vi "GLdrv_TRIG_COND_SOUR.vi"(0 "Connection ID":T2, 5 "COND":i32=1 min=0 max=1, 7 "Source":T1(ring), 9 "Alarm Time or Date":string, 11 "error in (no error)":errorcluster, 12 "Week":u8 format="%08b", 13 "Query(f)":bool) -> (4 "Connection ID Out":T2, 8 "Source out":T1(ring), 10 "Alarm Time or Date out":string, 14 "Week out":u8 format="%08b", 15 "error out":errorcluster)   [LabVIEW 2017, in "GL860_Driver.lvlib"]
doc: "トリガを検知する種類を設定します\nOff：　トリガを検知しません\nAMP: 指定ﾚﾍﾞﾙでトリガを検知します(CH,LOGIC,PULSEで設定)\nALAR：　アラーム発生でトリガを検知します。\nDATE：　指定時刻でトリガを検知します。(繰り返しOFF時に有効です)\n例）:TRIG:COND0:DATE,\"2010-01-01 00:00:00”\nLDATE：　指定時間でトリガを検知します。(繰り返しON時に有効です)\n例）:TRIG:COND1:LDATE,\"12:34:56”\nWEEK: 曜日と時間でトリガを検知します。\n<曜日設定> ０１２３４５６７ (8bit) 0=Off/1=On\n日月火水木金土\n例）　:TRIG:COND0:SOUR WEEK,127,\"12:34:56”\nEXTernal: 外部信号でトリガを検知します\nTIME: 時間経過(秒)でトリガを検知します(指定時間経過したら開始ま\nたは停止します。）\n例）　:TRIG:COND1:SOUR TIME,6000 (ストップトリガを100分後に設\n定します)"
uses:
  GL860_Driver.lvlib
  ConnectionID.ctl
  GLdrv_RW.ctl
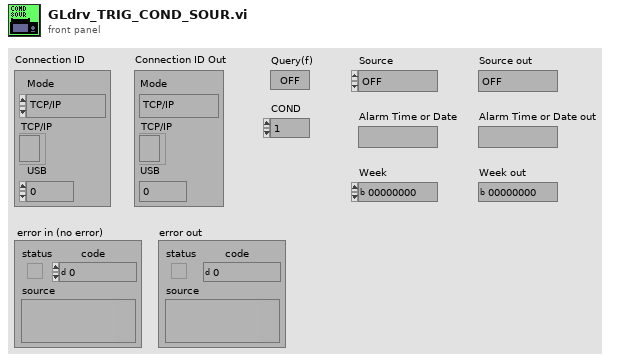
[diagram p1: front panel]
types:
  T1 = enum16{"OFF", "AMP", "ALAR", "DATE", "LDATE", "WEEK", "EXT", "TIME"}
  T2 = typedef "ConnectionID.ctl" = cluster{"Mode":enum16{"TCP/IP", "USB"}, "TCP/IP":refnum<k5>, "USB":i32}
  T3 = typedef "GLdrv_RW.ctl" = enum16{"Auto", "Read", "Write", "Buffer"}
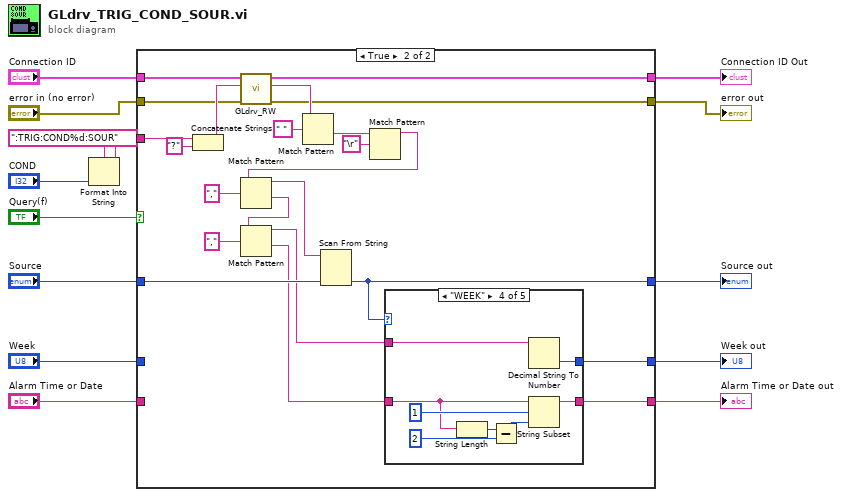
[diagram p0: block diagram]
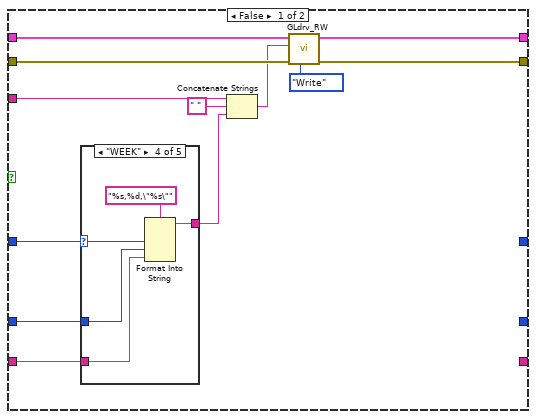
[diagram p2: hidden frame]
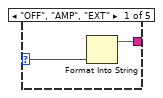
[diagram p3: hidden frame]
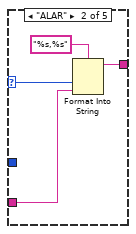
[diagram p4: hidden frame]
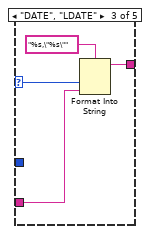
[diagram p5: hidden frame]
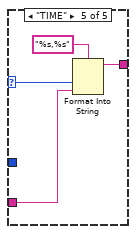
[diagram p6: hidden frame]
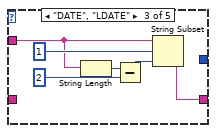
[diagram p9: hidden frame]
diagram:
  n1 = Format Into String(format string=":TRIG:COND%d:SOUR" ("Command"), "COND") -> (resulting string=w9:string)  [unwired: 2 in, 1 out]
  n2 = case shown="TRUE" "Query(f)" {
    tunnel: w9 -> [w26 w64]
    tunnel: [w21 w57] -> w14
    tunnel: [w23 w61] -> w13
    tunnel: "Connection ID" -> [w24 w62]
    tunnel: "error in (no error)" -> [w22 w58]
    tunnel: "Source" -> [w15 w56]
    tunnel: [_ w50] -> w6
    tunnel: "Alarm Time or Date" -> [w17 _]
    tunnel: "Week" -> [w16 _]
    tunnel: [_ w49] -> w3
    tunnel: [_ w47] -> w2
    frame False {
      n3 = case shown="\"WEEK\"" w15 {
        selector: w15 -> [w27 w31 w35 w40 w44]
        tunnel: [w28 w32 w36 w41 w45] -> w18
        tunnel: w17 -> [_ w29 w33 w38 w42]
        tunnel: w16 -> [_ _ _ w37 _]
        frame "OFF", "AMP", "EXT" {
          n4 = Format Into String(w27) -> (resulting string=w28:string)  [unwired: 3 in, 1 out]
        }
        frame "ALAR" {
          n5 = Format Into String(format string="%s,%s", w31, w29) -> (resulting string=w32:string)  [unwired: 2 in, 1 out]
        }
        frame "DATE", "LDATE" {
          n6 = Format Into String(format string="%s,\"%s\"", w35, w33) -> (resulting string=w36:string)  [unwired: 2 in, 1 out]
        }
        frame "WEEK" {
          n7 = Format Into String(format string="%s,%d,\"%s\"", w40, w37, w38) -> (resulting string=w41:string)  [unwired: 2 in, 1 out]
        }
        frame "TIME" {
          n8 = Format Into String(format string="%s,%s", w44, w42) -> (resulting string=w45:string)  [unwired: 2 in, 1 out]
        }
      }
      n9 = Concatenate Strings(w26, " " ("string"), w18) -> (w20:string)
      n10 = call "GLdrv_RW.vi"("Mode(read)"=GLdrv_RW."Write", "error in (no error)"=w22, "data in"=w20, "Connection ID"=w24) -> ("error out"=w21:errorcluster, "Connection ID Out"=w23:T2)  [unwired: 3 in, 3 out]
    }
    frame True {
      n11 = Concatenate Strings(w64, "?" ("string")) -> (w60:string)
      n12 = call "GLdrv_RW.vi"("error in (no error)"=w58, "data in"=w60, "Connection ID"=w62) -> ("error out"=w57:errorcluster, "data out"=w59:string, "Connection ID Out"=w61:T2)  [unwired: 4 in, 2 out]
      n13 = Match Pattern(string=w59, regular expression=" " ("search string/char (-)")) -> (after substring=w65:string)  [unwired: 4 out]
      n14 = Match Pattern(string=w65, regular expression="\r") -> (before substring=w53:string)  [unwired: 4 out]
      n15 = Match Pattern(string=w53, regular expression=",") -> (before substring=w51:string, after substring=w52:string)  [unwired: 3 out]
      n16 = Match Pattern(string=w52, regular expression=",") -> (before substring=w48:string, after substring=w46:string)  [unwired: 3 out]
      n17 = Scan From String(input string=w51, default 1=w56) -> (output 1=w50:T1)  [unwired: 3 in, 3 out]
      n18 = case shown="\"WEEK\"" w50 {
        tunnel: [_ w68 w69 w77 w83] -> w49
        tunnel: w48 -> [_ w68 w70 w76 w83]
        tunnel: [_ _ _ w75 _] -> w47
        tunnel: w46 -> [_ _ _ w78 _]
        frame "OFF", "AMP", "EXT" {
        }
        frame "ALAR" {
        }
        frame "DATE", "LDATE" {
          n19 = String Length(string=w70) -> (length=w73:i32)
          n20 = Subtract(x=w73, y=2) -> (x-y=w72:i32)
          n21 = String Subset(string=w70, offset (0)=1, length (rest)=w72) -> (substring=w69:string)
        }
        frame "WEEK" {
          n22 = String Length(string=w78) -> (length=w81:i32)
          n23 = Subtract(x=w81, y=2) -> (x-y=w80:i32)
          n24 = Decimal String To Number(string=w76) -> (number=w75:i32)  [unwired: 3 out]
          n25 = String Subset(string=w78, offset (0)=1, length (rest)=w80) -> (substring=w77:string)
        }
        frame "TIME" {
        }
      }
    }
  }
  "Connection ID Out" <- w13
  "error out" <- w14
  "Source out" <- w6
  "Alarm Time or Date out" <- w3
  "Week out" <- w2
